vi "Rename Engine to Match Bus.vi"(8 "error in (no error)":errorcluster, 9 "Current Bus Number":i32, 10 "Path to File":string="SPIEngineSOM.vi", 11 "Current Bus Path":path) -> (0 "error out":errorcluster, 3 "New File Path":path)   [LabVIEW 2014, in "Initialization and IO Node Scripting.lvlib"]
uses:
  Initialization and IO Node Scripting.lvlib
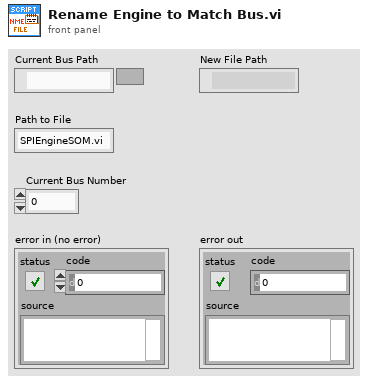
[diagram p1: front panel]
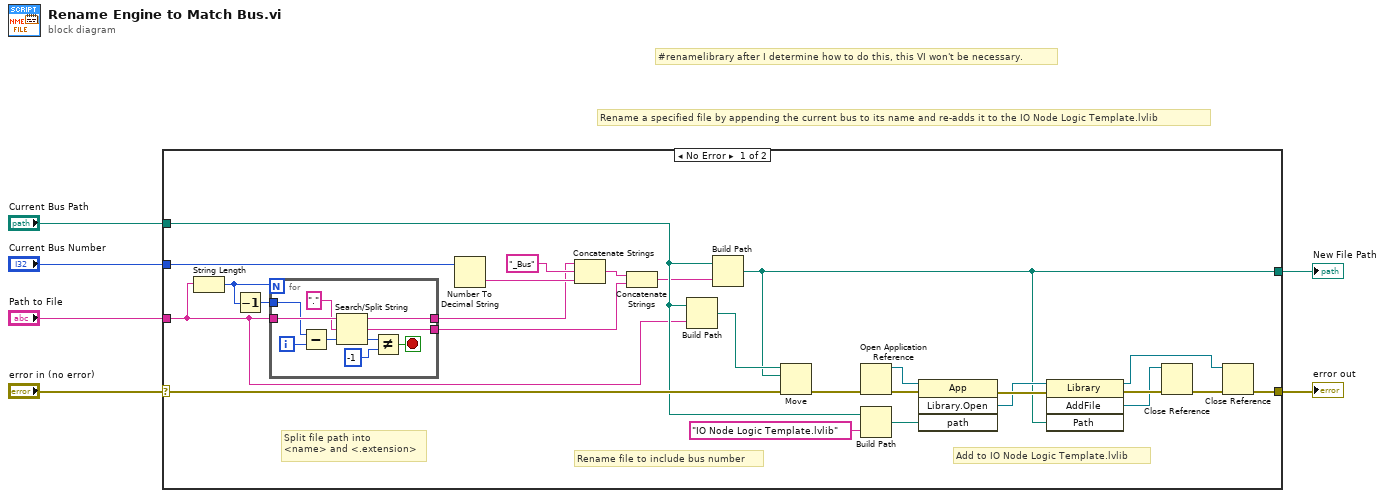
[diagram p0: block diagram]
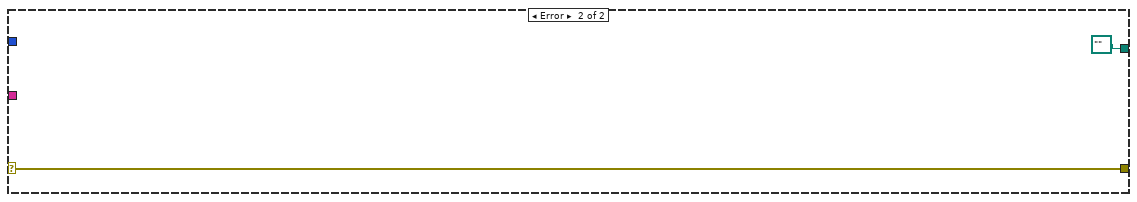
[diagram p2: hidden frame]
diagram:
  # "#renamelibrary after I determine how to do this, this VI won't be necessary."
  # "Rename a specified file by appending the current bus to its name and re-adds it to the IO Node Logic Template.lvlib"
  n1 = case shown="No Error" "error in (no error)" {
    selector: "error in (no error)" -> [w32 w44]
    tunnel: "Current Bus Path" -> [w15 _]
    tunnel: "Current Bus Number" -> [w31 _]
    tunnel: [w20 w44] -> w3
    tunnel: "Path to File" -> [w11 _]
    tunnel: [w17 path "" ("appended path")] -> w1
    frame No Error {
      # "Split file path into \n<name> and <.extension>"
      # "Add to IO Node Logic Template.lvlib"
      # "Rename file to include bus number"
      n2 = String Length(string=w11) -> (length=w13:i32)
      n3 = Decrement(x=w13) -> (x-1=w12:i32)
      n4 = for {
        N: w13 -> [_]
        tunnel: w11 -> [w42]
        tunnel: w12 -> [w37]
        tunnel: [w35] -> w7
        tunnel: [w34] -> w8
        i -> [w36]
        stop <- w39 stop-if-true
        n5 = Subtract(x=w37, y=w36) -> (x-y=w38:i32)
        n6 = Search/Split String(string=w42, search string/char (-)=".", offset (0)=w38) -> (substring before match=w35:string, match + rest of string=w34:string, offset of match=w41:i32)
        n7 = Not Equal?(x=w41, y=-1) -> (x != y?=w39:bool)
      }
      n8 = Number To Decimal String(number=w31) -> (decimal integer string=w30:string)  [unwired: 1 in]
      n9 = Concatenate Strings(w7, "_Bus" ("string"), w30) -> (w10:string)
      n10 = Concatenate Strings(w10, w8) -> (w9:string)
      n11 = Build Path(base path=w15, name or relative path=w11) -> (appended path=w28:path)
      n12 = Build Path(base path=w15, name or relative path=w9) -> (appended path=w17:path)
      n13 = Move(source path=w28, error in=w32, 10:w17) -> (error out=w27:errorcluster)  [unwired: 2 in, 2 out]
      n14 = Open Application Reference(8:w27) -> (0:w25:errorcluster, 3:w26:refnum<vi>)  [unwired: 3 in]
      n15 = Build Path(base path=w15, name or relative path="IO Node Logic Template.lvlib") -> (appended path=w16:path)
      n16 = invoke class="App" method="Library.Open"(reference=w26, error in=w25, "path"=w16) -> (error out=w24:errorcluster, "Open Library"=w23:refnum<vi>)  [unwired: 1 in, 2 out]
      n17 = invoke class="Library" method="AddFile"(reference=w23, error in=w24, "Path"=w17) -> (reference out=w18:refnum<vi>, error out=w21:errorcluster, "AddFile"=w19:refnum<vi>)  [unwired: 1 in, 1 out]
      n18 = Close Reference(reference=w19, error in (no error)=w21) -> (error out=w22:errorcluster)
      n19 = Close Reference(reference=w18, error in (no error)=w22) -> (error out=w20:errorcluster)
    }
    frame Error {
    }
  }
  "error out" <- w3
  "New File Path" <- w1
